vi "control_target.vi"() -> ()   [LabVIEW 2011]
uses:
  controls.llb/RTFIFO operate.ctl
  controls.llb/RTFIFO name.ctl
  <vilib>/DAQmx/create/channels.llb/DAQmx Create Channel (DI-Digital Input).vi
  <vilib>/DAQmx/read.llb/DAQmx Read (Digital U32 1Chan 1Samp).vi
panel:
  in  "Cluster":T1={"task"="", "error"={"status"=FALSE, "code"=0, "source"=""}, "Port"="PXI2Slot10/port0_24"}
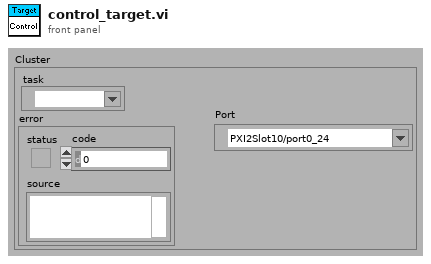
[diagram p1: front panel]
types:
  T1 = cluster{"task":refnum<k21>, "error":errorcluster, "Port":tag}
  T2 = typedef "RTFIFO operate.ctl" = enum16{"Creat", "Write", "Read", "Delete"}
  T3 = typedef "RTFIFO name.ctl" = enum16{"command_daq", "command_control", "data for save", "data for host", "dev status", "status for save"}
  T4 = typedef "data from RTFIFO.ctl" = cluster{"data for save":dbl[][], "data for host":dbl[][], "command_daq":u16, "command_control":u16, "dev status":u16[][], "status for save":u16[][]}
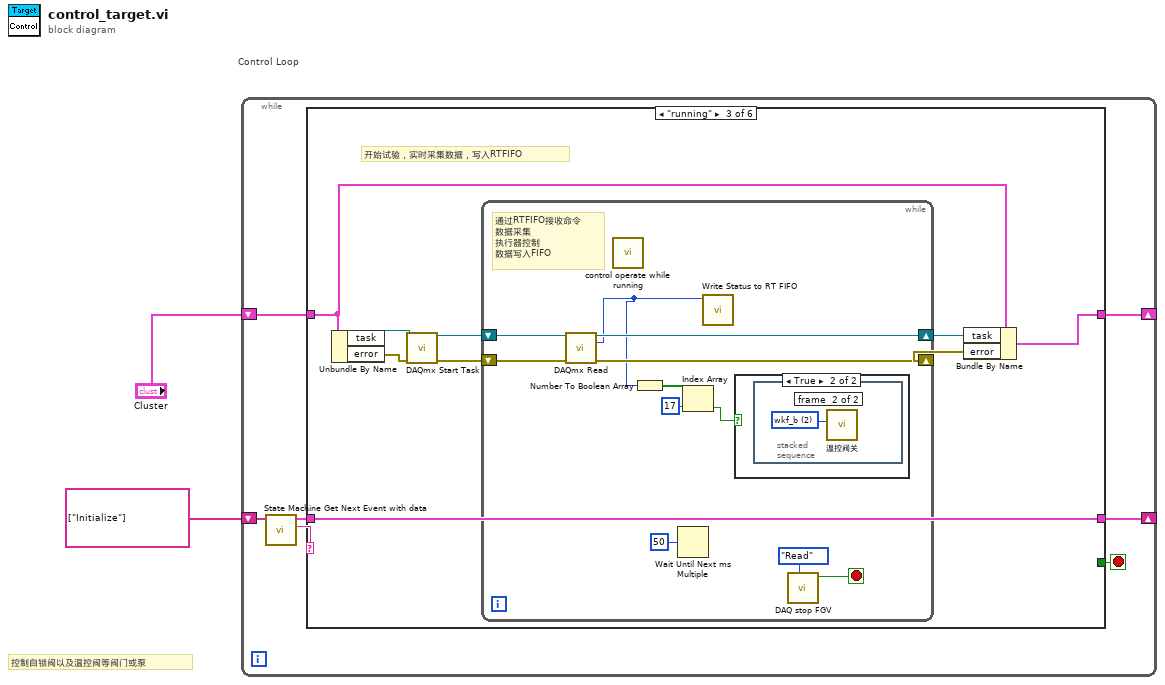
[diagram p0: block diagram]
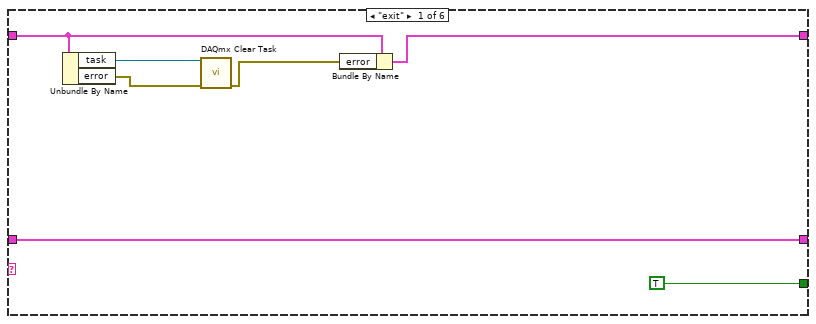
[diagram p2: hidden frame]
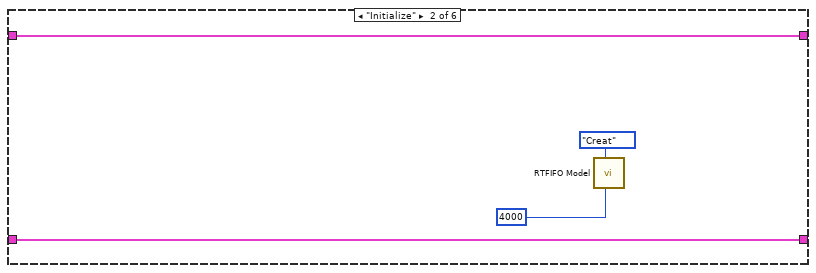
[diagram p3: hidden frame]
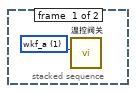
[diagram p5: hidden frame]
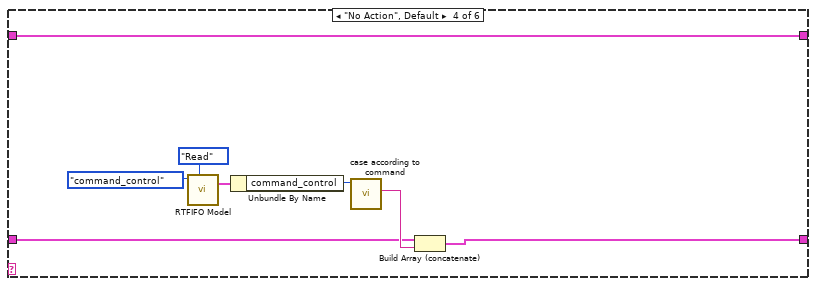
[diagram p6: hidden frame]
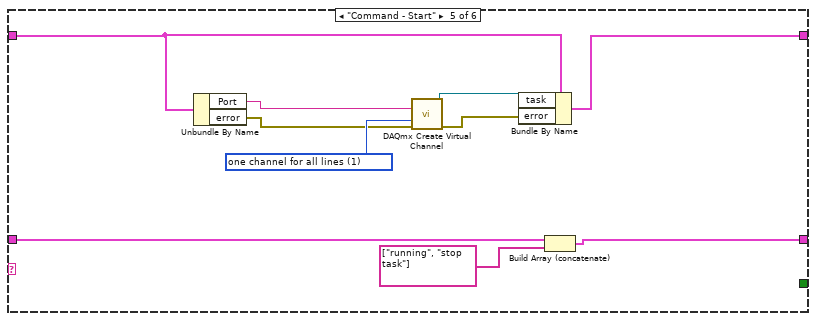
[diagram p7: hidden frame]
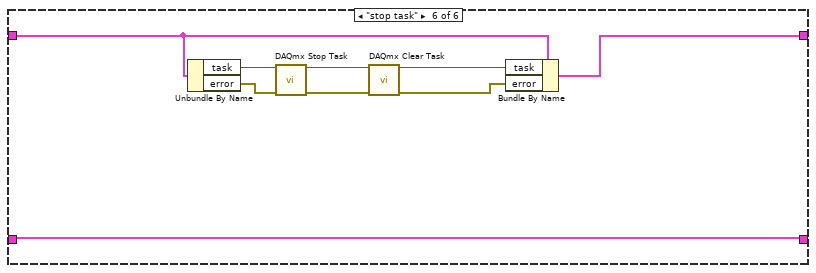
[diagram p8: hidden frame]
diagram:
  # "控制自锁阀以及温控阀等阀门或泵"
  # "Control Loop"
  n1 = while {
    shift-right: [w6] -> _
    shift-left: string[] ["Initialize"] -> [w9]
    shift-right: [w3] -> _
    shift-left: "Cluster" -> [w4]
    stop <- w5 stop-if-true
    n2 = call "State Machine Get Next Event with data.vi"("enent data queue in"=w9) -> ("next event"=w8:string, "event queue out"=w7:cluster{"event":string, "data":string}[])  [unwired: 5 in]
    n3 = case shown="\"running\"" w8 {
      tunnel: w7 -> [w16 w18 w21 w44 w53 w64]
      tunnel: [w16 w18 w21 w43 w52 w64] -> w6
      tunnel: [TRUE _ _ _ _ _] -> w5
      tunnel: w4 -> [w12 w17 w25 w50 w56 w66]
      tunnel: [w10 w17 w22 w50 w55 w65] -> w3
      frame "exit" {
        n4 = Unbundle By Name(w12) -> ("task"=w14:refnum<k21>, "error"=w13:errorcluster)
        n5 = call <vilib>:"DAQmx Clear Task.vi"("task in"=w14, "error in"=w13) -> ("error out"=w11:errorcluster)  [unwired: 13 in]
        n6 = Bundle By Name(cluster=w12, "error"=w11) -> (w10:T1)
      }
      frame "Initialize" {
        n7 = call "RTFIFO Model.vi"("size"=4000, "operate"=RTFIFO_operate."Creat") -> ()  [unwired: 8 in, 2 out]
      }
      frame "running" {
        # "开始试验，实时采集数据，写入RTFIFO"
        n8 = Unbundle By Name(w25) -> ("task"=w29:refnum<k21>, "error"=w28:errorcluster)
        n9 = call <vilib>:"DAQmx Start Task.vi"("task/channels in"=w29, "error in"=w28) -> ("task out"=w27:refnum<k21>, "error out"=w26:errorcluster)  [unwired: 12 in]
        n10 = while {
          shift-right: [w37] -> w24
          shift-left: w27 -> [w40]
          shift-right: [w38] -> w23
          shift-left: w26 -> [w39]
          stop <- w35 stop-if-true
          # "通过RTFIFO接收命令\n数据采集\n执行器控制\n数据写入FIFO"
          n11 = call-poly <vilib>:"DAQmx Read.vi"("task/channels in"=w40, "error in"=w39) -> ("task out"=w37:refnum<k21>, "data"=w33:u32, "error out"=w38:errorcluster)  [unwired: 11 in]
          n12 = call "control operate while running.vi"() -> ()  [unwired: 1 in]
          n13 = Number To Boolean Array(number=w33) -> (Boolean array=w32:bool[])
          n14 = Wait Until Next ms Multiple(millisecond multiple=u32 50) -> ()  [unwired: 1 out]
          n15 = Index Array(array=w32, index=17) -> (element=w30:bool)
          n16 = call "Write Status to RT FIFO.vi"("status"=w33) -> ()  [unwired: 11 in]
          n17 = case shown="True" w30 {
            frame False {
            }
            frame True {
              n18 = stacked-sequence {
                frame #0 {
                  w41 = u16 1 items=["Default", "wkf_a", "wkf_b"] ("温控阀名称")
                  n19 = call "温控阀关.vi"("温控阀名称"=w41) -> ()  [unwired: 10 in, 1 out]
                }
                frame #1 {
                  w42 = u16 2 items=["Default", "wkf_a", "wkf_b"] ("温控阀名称")
                  n20 = call "温控阀关.vi"("温控阀名称"=w42) -> ()  [unwired: 10 in, 1 out]
                }
              }
            }
          }
          n21 = call "DAQ stop FGV.vi"("W/R"=enum16{"Read", "Write"}."Read") -> ("stop ?"=w35:bool)  [unwired: 10 in]
        }
        n22 = Bundle By Name(cluster=w25, "task"=w24, "error"=w23) -> (w22:T1)
      }
      frame "No Action", Default {
        n23 = call "RTFIFO Model.vi"("operate"=RTFIFO_operate."Read", "FIFO name"=RTFIFO_name."command_control") -> ("data"=w47:T4)  [unwired: 8 in, 1 out]
        n24 = Unbundle By Name(w47) -> ("command_control"=w46:u16)
        n25 = call "case according to command.vi"("command"=w46) -> ("case"=w45:string)  [unwired: 9 in, 1 out]
        n26 = Build Array (concatenate)(w44, w45) -> (w43:cluster{"event":string, "data":string}[])
      }
      frame "Command - Start" {
        w60 = 1 items=["one channel for each line", "one channel for all lines"] ("line grouping")
        n27 = Unbundle By Name(w56) -> ("Port"=w51:tag, "error"=w59:errorcluster)
        n28 = call-poly <vilib>:"DAQmx Create Virtual Channel.vi"("lines"=w51, "line grouping"=w60, "error in"=w59) -> ("task out"=w58:refnum<k21>, "error out"=w57:errorcluster)  [unwired: 11 in]
        n29 = Bundle By Name(cluster=w56, "task"=w58, "error"=w57) -> (w55:T1)
        n30 = Build Array (concatenate)(w53, string[] ["running", "stop task"] ("element")) -> (w52:cluster{"event":string, "data":string}[])
      }
      frame "stop task" {
        n31 = Unbundle By Name(w66) -> ("task"=w68:refnum<k21>, "error"=w67:errorcluster)
        n32 = call <vilib>:"DAQmx Stop Task.vi"("task/channels in"=w68, "error in"=w67) -> ("task out"=w63:refnum<k21>, "error out"=w62:errorcluster)  [unwired: 12 in]
        n33 = call <vilib>:"DAQmx Clear Task.vi"("task in"=w63, "error in"=w62) -> ("error out"=w61:errorcluster)  [unwired: 13 in]
        n34 = Bundle By Name(cluster=w66, "task"=w63, "error"=w61) -> (w65:T1)
      }
    }
  }
